vi "Prax13y1.vi"() -> ()   [LabVIEW 2020]
panel:
  out "x-y 2":u32
  out "x-y":u32
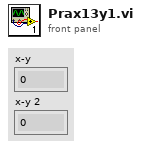
[diagram p1: front panel]
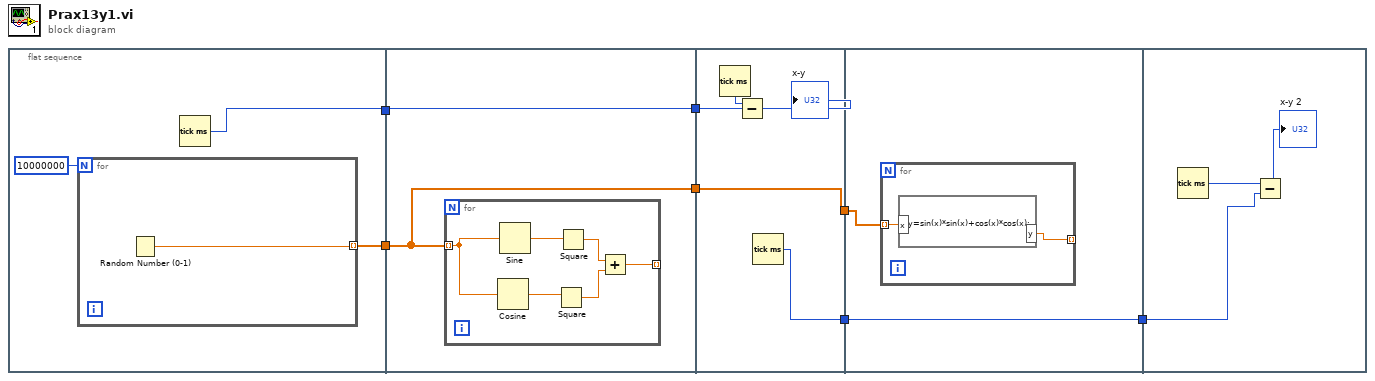
[diagram p0: block diagram]
diagram:
  n1 = flat-sequence {
    tunnel: [w10] -> w7
    tunnel: [w8] -> w5
    tunnel: w7 -> [w13]
    tunnel: [w13] -> w6
    tunnel: w5 -> [w12]
    tunnel: [w12] -> w4
    tunnel: w6 -> [w23]
    tunnel: w4 -> [w21]
    tunnel: [w21] -> w3
    tunnel: [w20] -> w2
    tunnel: w3 -> [w26]
    tunnel: w2 -> [w25]
    tunnel: [w25] -> w1
    tunnel: w1 -> [w30]
    frame #0 {
      n2 = for {
        N: 10000000 -> [_]
        tunnel: [w11] -> w8 mode=indexing
        n3 = Random Number (0-1)() -> (number: 0 to 1=w11:dbl)
      }
      n4 = Tick Count (ms)() -> (millisecond timer value=w10:u32)
    }
    frame #1 {
      n5 = for {
        tunnel: w12 -> [w19] mode=indexing
        tunnel: [w14] -> _ mode=indexing
        n6 = Cosine(x=w19) -> (cos(x)=w17:dbl)
        n7 = Sine(x=w19) -> (sin(x)=w18:dbl)
        n8 = Square(x=w17) -> (x^2=w15:dbl)
        n9 = Square(x=w18) -> (x^2=w16:dbl)
        n10 = Add(x=w16, y=w15) -> (x+y=w14:dbl)
      }
    }
    frame #2 {
      n11 = Tick Count (ms)() -> (millisecond timer value=w24:u32)
      n12 = Subtract(x=w24, y=w23) -> (x-y=→"x-y":u32)
      n13 = Tick Count (ms)() -> (millisecond timer value=w20:u32)
    }
    frame #3 {
      n14 = for {
        tunnel: w26 -> [w28] mode=indexing
        tunnel: [w27] -> _ mode=indexing
        n15 = formula code="y=sin(x)*sin(x)+cos(x)*cos(x);"("x"=w28) -> ("y"=w27:dbl)
      }
    }
    frame #4 {
      n16 = Tick Count (ms)() -> (millisecond timer value=w29:u32)
      n17 = Subtract(x=w29, y=w30) -> (x-y=→"x-y 2":u32)
    }
  }
